vi "G# - SerializationExample.vi"() -> ()   [LabVIEW 2017]
doc: "Serialization\nThis example serializes an object as binary or xml string. A new object is then created and deserialized from the stored state of the previous object.\n\nBy using the G# Debugger found in Tools->G# Debugger a text log can be followed showing how the objects were created and destroyed."
uses:
  MyTestClass_class/MyTestClass.lvclass
  <vilib>/addons/_AddQ/G#Object/G#Object.lvclass
panel:
  in  "error in (no error)":errorcluster
  in  "as xml":bool
  out "City out":string
  out "Address out":string
  out "Name out":string
  out "error out":errorcluster
  in  "City":string="Stockholm"
  in  "Address":string="Royal Castle"
  in  "Name":string="Carl XVI Gustav"
  # "Serialization\nThis example serializes an object as binary or xml string.\nA new object is then created and deserialized from the stored state of the previous object.\n\nBy using the G# Debugger found in Tools->G# Debugger a text log can be followed showing how the objects were created and destroyed."
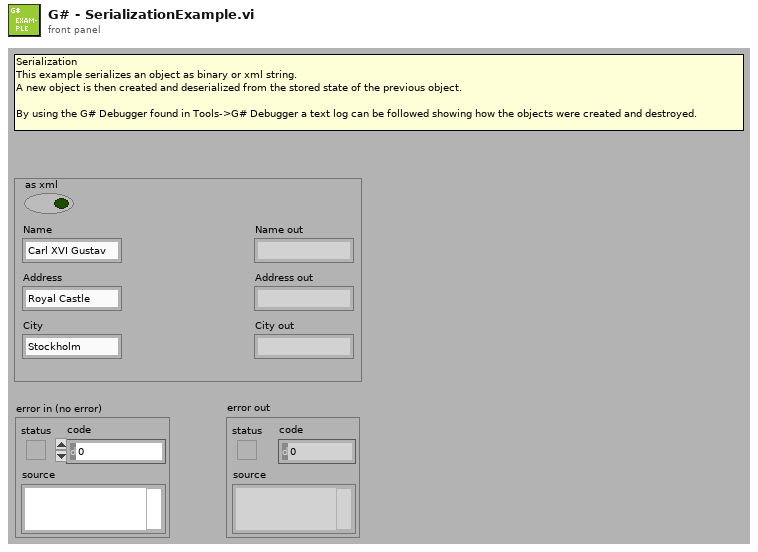
[diagram p1: front panel]
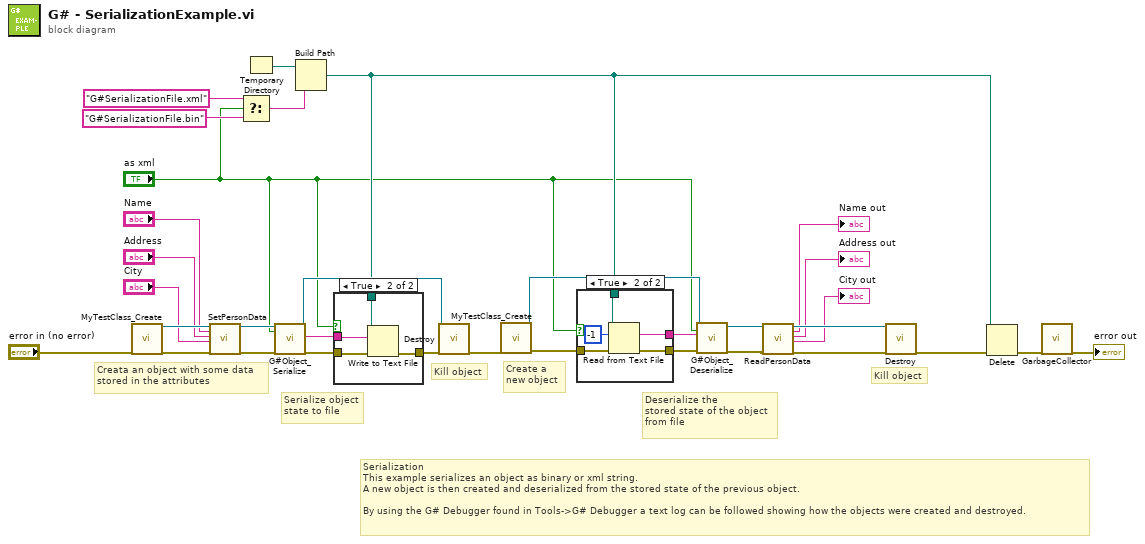
[diagram p0: block diagram]
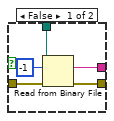
[diagram p2: hidden frame]
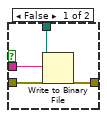
[diagram p3: hidden frame]
diagram:
  # "Serialization\nThis example serializes an object as binary or xml string.\nA new object is then created and deserialized from the stored state of the previous object.\n\nBy using the G# Debugger found in Tools->G# Debugger a text log can be followed showing how the objects were created and destroyed."
  # "Kill object"
  # "Deserialize the\nstored state of the object\nfrom file"
  # "Create a\nnew object"
  # "Kill object"
  # "Serialize object\nstate to file"
  # "Creata an object with some data\nstored in the attributes"
  n1 = call "MyTestClass_Create.vi"("error in (no error)"="error in (no error)") -> ("reference out"=w32:refnum<class "MyTestClass.lvclass">, "error out"=w33:errorcluster)  [unwired: 17 in]
  n2 = call-dynamic "SetPersonData.vi"("reference in"=w32, "Name"="Name", "Address"="Address", "City"="City", "error in (no error)"=w33) -> ("reference out"=w25:refnum<class "MyTestClass.lvclass">, "error out"=w26:errorcluster)  [unwired: 13 in]
  n3 = Select(t="G#SerializationFile.xml" ("name or relative path"), s="as xml", f="G#SerializationFile.bin" ("name or relative path")) -> (s? t:f=w2:string)
  n4 = Temporary Directory() -> (w21:path)
  n5 = call-dynamic "G#Object_Serialize.vi"("reference in"=w25, "as xml (F)"="as xml", "error in (no error)"=w26) -> ("reference out"=w31:refnum<class "MyTestClass.lvclass">, "serialized object"=w22:string, "error out"=w24:errorcluster)  [unwired: 13 in, 1 out]
  n6 = Build Path(base path=w21, name or relative path=w2) -> (appended path=w5:path)
  n7 = case shown="True" "as xml" {
    tunnel: w24 -> [w37 w41]
    tunnel: [w36 w39] -> w23
    tunnel: w22 -> [w35 w40]
    tunnel: w5 -> [w34 w38]
    frame False {
      n8 = Write to Binary File(file (use dialog)=w34, data=w35, error in=w37) -> (error out=w36:errorcluster)  [unwired: 3 in, 2 out]
    }
    frame True {
      n9 = Write to Text File(file (use dialog)=w38, text=w40, error in=w41) -> (error out=w39:errorcluster)  [unwired: 1 in, 2 out]
    }
  }
  n10 = call-dynamic "Destroy.vi"("reference in"=w31, "error in (no error)"=w23) -> ("error out"=w20:errorcluster)  [unwired: 16 in, 1 out]
  n11 = call "MyTestClass_Create.vi"("error in (no error)"=w20) -> ("reference out"=w19:refnum<class "MyTestClass.lvclass">, "error out"=w18:errorcluster)  [unwired: 17 in]
  n12 = case shown="True" "as xml" {
    tunnel: w18 -> [w46 w51]
    tunnel: [w44 w49] -> w17
    tunnel: [w43 w50] -> w16
    tunnel: w5 -> [w42 w47]
    frame False {
      n13 = Read from Binary File(8:w46, 10:-1 ("count (1)"), 11:w42) -> (0:w43:errorcluster, 2:w44:string)  [unwired: 3 in, 2 out]
    }
    frame True {
      n14 = Read from Text File(file (use dialog)=w47, count=-1, error in=w51) -> (text=w49:string, error out=w50:errorcluster)  [unwired: 1 in, 2 out]
    }
  }
  n15 = call-dynamic "G#Object_Deserialize.vi"("reference in"=w19, "as xml (F)"="as xml", "serialized object"=w17, "error in (no error)"=w16) -> ("reference out"=w14:refnum<class "MyTestClass.lvclass">, "error out"=w15:errorcluster)  [unwired: 13 in, 1 out]
  n16 = call-dynamic "ReadPersonData.vi"("reference in"=w14, "error in (no error)"=w15) -> ("reference out"=w12:refnum<class "MyTestClass.lvclass">, "Name"=→"Name out":string, "Address"=→"Address out":string, "City"=→"City out":string, "error out"=w13:errorcluster)  [unwired: 13 in]
  n17 = call-dynamic "Destroy.vi"("reference in"=w12, "error in (no error)"=w13) -> ("error out"=w8:errorcluster)  [unwired: 16 in, 1 out]
  n18 = Delete(path (use dialog)=w5, error in=w8) -> (error out=w7:errorcluster)  [unwired: 3 in, 2 out]
  n19 = call <vilib>:"GarbageCollector.vi"("error in (no error)"=w7) -> ("error out"=→"error out":errorcluster)  [unwired: 16 in, 2 out]
